vi "Msg.vi"(7 "Actor in":refnum<class "Actor.lvclass">, 11 "TEMPLATE Msg in":refnum<class "TEMPLATE Msg.lvclass">) -> (5 "Actor out":refnum<class "Actor.lvclass">)   [LabVIEW 2020, in "_Template.lvlib" / "Templates.lvlib" / "TEMPLATE Msg.lvlib" / "TEMPLATE Msg.lvclass"]
uses:
  TEMPLATE Msg.lvclass
  TEMPLATE/TEMPLATE.lvclass
  jettl/jettl/Actor/Actor/Actor.lvclass
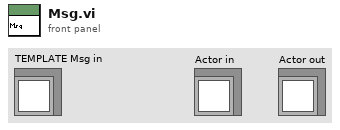
[diagram p1: front panel]
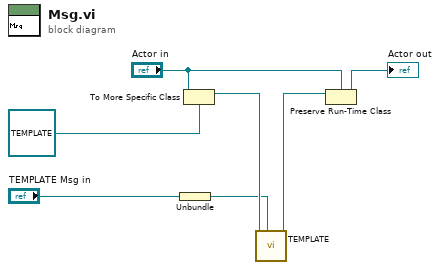
[diagram p0: block diagram]
diagram:
  n1 = Unbundle "Unbundle"("TEMPLATE Msg in") -> (w3:refnum<class "Sender.lvclass">)
  n2 = To More Specific Class(target class=refnum<class "TEMPLATE.lvclass"> refnum ("jettl Msg Template"), reference="Actor in") -> (specific class reference=w5:refnum<class "TEMPLATE.lvclass">)  [unwired: 1 in, 1 out]
  n3 = call-dynamic "TEMPLATE.vi"("Sender"=w3, "TEMPLATE in"=w5) -> ("TEMPLATE out"=w4:refnum<class "TEMPLATE.lvclass">)  [unwired: 9 in]
  n4 = Preserve Run-Time Class(object in=w4, 2:"Actor in") -> (object out=→"Actor out":refnum<class "Actor.lvclass">)  [unwired: 1 in, 1 out]
